vi "Cycle.vi"(8 "error in (no error)":errorcluster, 11 "FlePhysEffExperiment In":refnum<class "FlePhysEffExperiment.lvclass">) -> (0 "error out":errorcluster, 3 "FlePhysEffExperiment Out":refnum<class "FlePhysEffExperiment.lvclass">)   [LabVIEW 2010]
uses:
  FlePhysEffExperiment.lvclass
panel:
  out "XY Graph":cluster{"horizontal":dbl[], "vertical":dbl[]}[](graph)
  out "ExperimentStats":T1
  in  "FixationRadius":dbl=50.0
  in  "RewardAmount":dbl=50.0
  in  "Timeouts":T2={"Intertrial"=1000.0, "AcquireFixation"=1000.0, "HoldFixation"=300.0, "DelayPeriod"=1000.0, "ResponsePeriod"=1000.0}
  in  "Eye Params":dbl[](array[numeric])
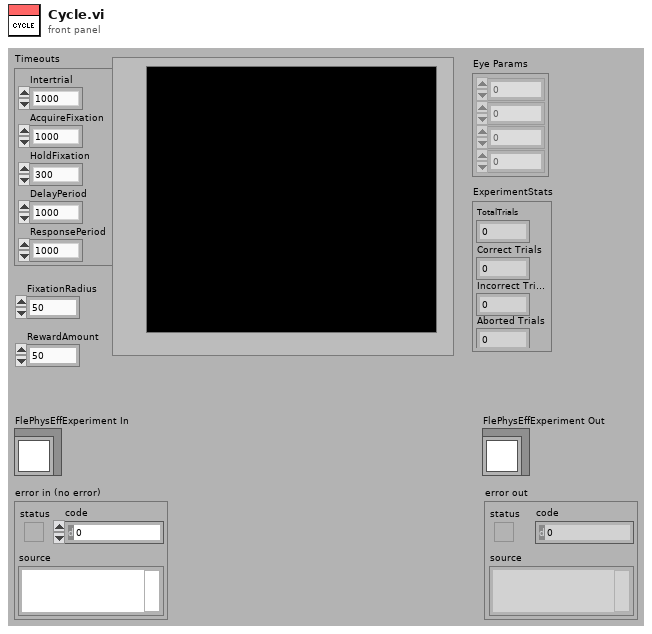
[diagram p1: front panel]
types:
  T1 = cluster{"TotalTrials":dbl, "Correct Trials":dbl, "Incorrect Trials":dbl, "Aborted Trials":dbl}
  T2 = cluster{"Intertrial":dbl, "AcquireFixation":dbl, "HoldFixation":dbl, "DelayPeriod":dbl, "ResponsePeriod":dbl}
  T3 = cluster{"TotalTrials":u32, "Correct Trials":u32, "Incorrect Trials":u32, "Aborted Trials":u32}
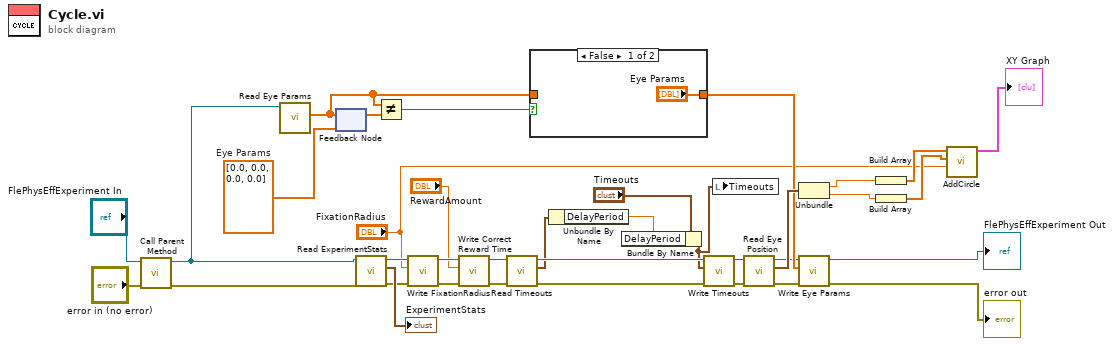
[diagram p0: block diagram]
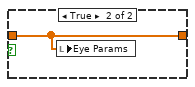
[diagram p2: hidden frame]
diagram:
  w29 = dbl[] [0.0, 0.0, 0.0, 0.0]  # Eye Params
  n1 = call-parent "Call Parent Method"("error in (no error)"="error in (no error)", "PassiveExperiment In"="FlePhysEffExperiment In") -> ("error out"=w20:errorcluster, "PassiveExperiment Out"=w15:refnum<class "FlePhysEffExperiment.lvclass">)  [unwired: 8 in]
  n2 = call-dynamic "Read Eye Params.vi"("TrialBasedExperiment in"=w15) -> ("Eye Params"=w30:dbl[])  [unwired: 8 in, 2 out]
  n3 = feedback #1(w29) -> (w27:dbl[])
  n4 = feedback-in #1(w30) -> ()
  n5 = call-dynamic "Read ExperimentStats.vi"("error in (no error)"=w20, "TrialBasedExperiment in"=w15) -> ("error out"=w22:errorcluster, "ExperimentStats"=→"ExperimentStats":T3, "TrialBasedExperiment out"=w21:refnum<class "FlePhysEffExperiment.lvclass">)  [unwired: 7 in]
  n6 = Not Equal?(x=w30, y=w27) -> (x != y?=w28:bool)
  n7 = call-dynamic "Write FixationRadius.vi"("error in (no error)"=w22, "FixationRadius"="FixationRadius", "MatlabExperiment in"=w21) -> ("error out"=w25:errorcluster, "MatlabExperiment out"=w24:refnum<class "FlePhysEffExperiment.lvclass">)  [unwired: 7 in]
  n8 = call-dynamic "Write Correct Reward Time.vi"("error in (no error)"=w25, "Correct Reward Time"="RewardAmount", "MatlabExperiment in"=w24) -> ("error out"=w2:errorcluster, "MatlabExperiment out"=w3:refnum<class "FlePhysEffExperiment.lvclass">)  [unwired: 7 in]
  n9 = call-dynamic "Read Timeouts.vi"("error in (no error)"=w2, "TrialBasedExperiment in"=w3) -> ("error out"=w7:errorcluster, "Timeouts"=w6:T2, "TrialBasedExperiment out"=w8:refnum<class "FlePhysEffExperiment.lvclass">)  [unwired: 7 in]
  n10 = case shown="False" w28 {
    tunnel: ["Eye Params" w38] -> w33
    tunnel: w30 -> [_ w38]
    frame False {
    }
    frame True {
      n11 = local write "Eye Params"(w38) -> ()
    }
  }
  n12 = Unbundle By Name(w6) -> ("DelayPeriod"=w4:dbl)
  n13 = Bundle By Name(cluster="Timeouts", "DelayPeriod"=w4) -> (w1:T2)
  n14 = call-dynamic "Write Timeouts.vi"("error in (no error)"=w7, "Timeouts"=w1, "TrialBasedExperiment in"=w8) -> ("error out"=w9:errorcluster, "TrialBasedExperiment out"=w10:refnum<class "FlePhysEffExperiment.lvclass">)  [unwired: 7 in]
  n15 = local write "Timeouts"(w1) -> ()
  n16 = call-dynamic "Read Eye Position.vi"("error in (no error)"=w9, "TrialBasedExperiment in"=w10) -> ("error out"=w32:errorcluster, "Eye Position"=w34:cluster{"Horizontal":dbl, "Vertical":dbl}, "TrialBasedExperiment out"=w31:refnum<class "FlePhysEffExperiment.lvclass">)  [unwired: 7 in]
  n17 = Unbundle(w34) -> ("Horizontal"=w19:dbl, "Vertical"=w18:dbl)
  n18 = call-dynamic "Write Eye Params.vi"("error in (no error)"=w32, "Eye Params"=w33, "TrialBasedExperiment in"=w31) -> ("error out"=→"error out":errorcluster, "TrialBasedExperiment out"=→"FlePhysEffExperiment Out":refnum<class "FlePhysEffExperiment.lvclass">)  [unwired: 7 in]
  n19 = Build Array(w19) -> (w14:dbl[])
  n20 = Build Array(w18) -> (w13:dbl[])
  n21 = call "AddCircle.vi"("radius"="FixationRadius", "vertical"=w13, "horizontal"=w14) -> ("output"=→"XY Graph":cluster{"horizontal":dbl[], "vertical":dbl[]}[])  [unwired: 8 in]
